vi "fft -- manipulate waveform -- V1.vi"(4 "range max":dbl=0.07527795000000001 format="%#_3p", 6 "range min":dbl=0.07527795000000001 format="%#_3p", 7 "fft -- manipulate":T1, 8 "time (sec)":dbl=0.07527795000000001 format="%#_3p", 11 "power spectra":cluster{"f0":dbl, "df":dbl, "magnitude":dbl[]}[](array[cluster]) {"magnitude" format="%.2p"; "f0" format="%.2p"; "df" format="%.2p"}) -> (0 "XY Graph":cluster{dbl[], dbl[]}(graph), 2 "F of max":dbl=0.011117700000000001 format="%#_8p", 3 "Amp of max":dbl=0.011117700000000001 format="%#_3p")   [LabVIEW 2021]
uses:
  fft -- manipulate waveform -- control.vi.ctl
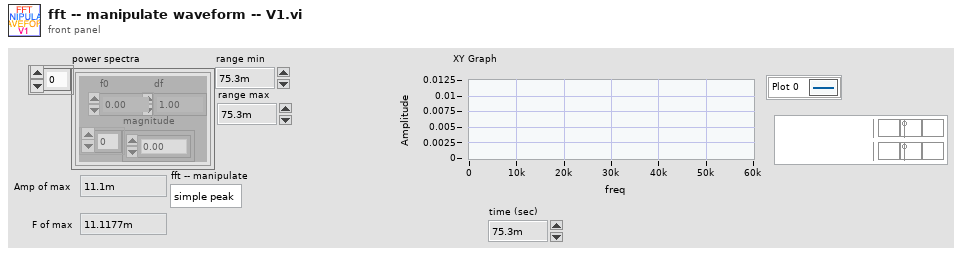
[diagram p1: front panel]
types:
  T1 = typedef "fft -- manipulate waveform -- control.vi.ctl" = enum16{"simple peak", "to array"}
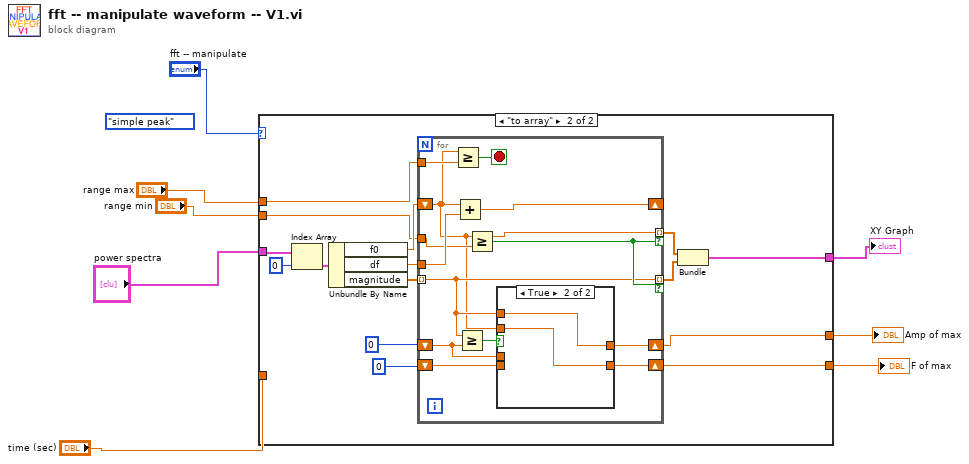
[diagram p0: block diagram]
diagram:
  (unwired) fft_--_manipulate_waveform_--_control.vi."simple peak" ("fft -- manipulate")
  n1 = case shown="\"to array\"" "fft -- manipulate" {
    tunnel: "power spectra" -> [_ w23]
    tunnel: "time (sec)" -> [_ _]
    tunnel: "range max" -> [_ w15]
    tunnel: "range min" -> [_ w14]
    tunnel: [_ w11] -> w6
    tunnel: [_ w10] -> w5
    tunnel: [_ w9] -> w1
    frame "simple peak", Default {
    }
    frame "to array" {
      n2 = Index Array(array=w23, index=0) -> (element=w21:cluster{"f0":dbl, "df":dbl, "magnitude":dbl[]})
      n3 = Unbundle By Name(w21) -> ("f0"=w19:dbl, "df"=w18:dbl, "magnitude"=w20:dbl[])
      n4 = for {
        tunnel: w20 -> [w27] mode=indexing
        tunnel: [w27] -> w16 mode=indexing if=w33
        shift-right: [w36] -> _
        shift-left: w19 -> [w25]
        tunnel: [w25] -> w17 mode=indexing if=w33
        tunnel: w18 -> [w35]
        tunnel: w15 -> [w32]
        tunnel: w14 -> [w31]
        shift-right: [w28] -> w11
        shift-left: i64 0 ("Start") -> [w29]
        shift-right: [w26] -> w10
        shift-left: i64 0 ("Start") -> [w24]
        stop <- w34 stop-if-true
        n5 = Greater Or Equal?(x=w25, y=w32) -> (x >= y?=w34:bool)
        n6 = Add(x=w25, y=w35) -> (x+y=w36:dbl)
        n7 = Greater Or Equal?(x=w27, y=w29) -> (x >= y?=w30:bool)
        n8 = Greater Or Equal?(x=w25, y=w31) -> (x >= y?=w33:bool)
        n9 = case shown="True" w30 {
          tunnel: w29 -> [w38 _]
          tunnel: [w38 w40] -> w28
          tunnel: w27 -> [_ w40]
          tunnel: [w37 w39] -> w26
          tunnel: w25 -> [_ w39]
          tunnel: w24 -> [w37 _]
          frame False {
          }
          frame True {
          }
        }
      }
      n10 = Bundle(w17, w16) -> (w9:cluster{dbl[], dbl[]})  [unwired: 1 in]
    }
  }
  "XY Graph" <- w1
  "Amp of max" <- w6
  "F of max" <- w5
